vi "Autonomous Independent.vi"   [LabVIEW 2017]
doc: "This VI is called when autonomous begins, and will automatically be terminated when autonomous ends. You can carry out timed or sensor driven robot movement independently without needing to return to the caller."
uses:
  <vilib>/Rock Robotics/WPI/Utilities/WPI_GetSetVariantRefNum.vi
  <vilib>/Rock Robotics/Network Tables/NT Write Numeric Array.vi
  <vilib>/Rock Robotics/Network Tables/NT Read String.vi
  <vilib>/Rock Robotics/WPI/RobotDrive/WPI_RobotDriveMecanumDrive_Cartesian.vi
types:
  T1 = typedef "WPI_JoystickDevRef.ctl" = cluster{"Device":T2}
  T2 = typedef "WPI_JoystickDeviceEnum.ctl" = enum16{"USB 0", "USB 1", "USB 2", "USB 3", "USB 4", "USB 5"}
  T3 = typedef "WPI_RobotDriveDevRef.ctl" = cluster{"DevStatus":errorcluster, "Motors[]":T4[], "Square Inputs":bool, "Max Output":dbl}
  T4 = typedef "WPI_MotorControlDeviceRef.ctl" = cluster{"DeviceStatus":errorcluster, "Type":T5, "PWM":cluster{"PWM Channel":T6, "DeadBand":T7}, "CAN":cluster{"Device Number":u8, "SetOutput VI Ref":variant, "GetOutput VI Ref":variant, "Enable VI Ref":variant, "Disable VI Ref":variant, "Data":variant}, "Invert":bool, "DIO PWM":cluster{"PWM \"Enable\" Channel":T6, "DIOChannel":T8, "PWM Rate":dbl}}
  T5 = typedef "WPI_MotorControlType.ctl" = enum16{"PWM", "CAN", "DIO PWM"}
  T6 = typedef "FPGA_DIOPWMChannel.ctl" = enum8{"PWM 0", "PWM 1", "PWM 2", "PWM 3", "PWM 4", "PWM 5", "PWM 6", "PWM 7", "PWM 8", "PWM 9", "PWM MXP 0", "PWM MXP 1", "PWM MXP 2", "PWM MXP 3", "PWM MXP 4", "PWM MXP 5", "PWM MXP 6", "PWM MXP 7", "PWM MXP 8", "PWM MXP 9", "Invalid"}
  T7 = typedef "WPI_PWMDeadband.ctl" = cluster{"Name":string, "maxPositivePwm":i32, "minPositivePwm":i32, "centerPwm":i32, "maxNegativePwm":i32, "minNegativePwm":i32, "angularRange":u16}
  T8 = typedef "FPGA_DIOChannel.ctl" = enum8{"DIO 0", "DIO 1", "DIO 2", "DIO 3", "DIO 4", "DIO 5", "DIO 6", "DIO 7", "DIO 8", "DIO 9", "DIO MXP 0", "DIO MXP 1", "DIO MXP 2", "DIO MXP 3", "DIO MXP 4", "DIO MXP 5", "DIO MXP 6", "DIO MXP 7", "DIO MXP 8", "DIO MXP 9", "DIO MXP 10", "DIO MXP 11", "DIO MXP 12", "DIO MXP 13", "DIO MXP 14", "DIO MXP 15", "SPI Port CS1", "SPI Port CS2", "SPI Port CS3", "SPI Port MISO", "SPI Port MOSI", "Invalid"}
  T9 = typedef "WPI_GyroDevRef.ctl" = cluster{"DevStatus":errorcluster, "Analog Channel":T10, "Gain (VoltsPerDegree/Second)":dbl, "Gyro Type":enum16{"Analog", "XRS450"}, "Handle":i32, "SPI Bus":T11, "Device Found":bool, "Sample Rate":dbl, "Calibrate On Open":bool, "Offset":dbl}
  T10 = typedef "FPGA_AIChannel.ctl" = enum8{"AI 0", "AI 1", "AI 2", "AI 3", "AI MXP 0", "AI MXP 1", "AI MXP 2", "AI MXP 3", "Invalid"}
  T11 = typedef "spi_bus.ctl" = enum16{"SPI On-Board, CS0", "SPI On-Board, CS1", "SPI On-Board, CS2", "SPI On-Board, CS3", "SPI MXP", "Invalid"}
  T12 = typedef "WPI_EncoderDevRef.ctl" = cluster{"DevStatus":errorcluster, "EncoderIndex":T13, "CounterIndex":T14, "DistancePerCount":dbl, "Decoding Type":T15}
  T13 = typedef "FPGA_EncoderIdx.ctl" = enum8{"Enc 0", "Enc 1", "Enc 2", "Enc 3", "Enc 4", "Enc 5", "Enc 6", "Enc 7", "Invalid"}
  T14 = typedef "FPGA_CounterCtrSystemIndex.ctl" = enum8{"Ctr 0", "Ctr 1", "Ctr 2", "Ctr 3", "Ctr 4", "Ctr 5", "Ctr 6", "Ctr 7", "Invalid"}
  T15 = typedef "WPI_EncoderType.ctl" = enum16{"1x", "2x", "4x"}
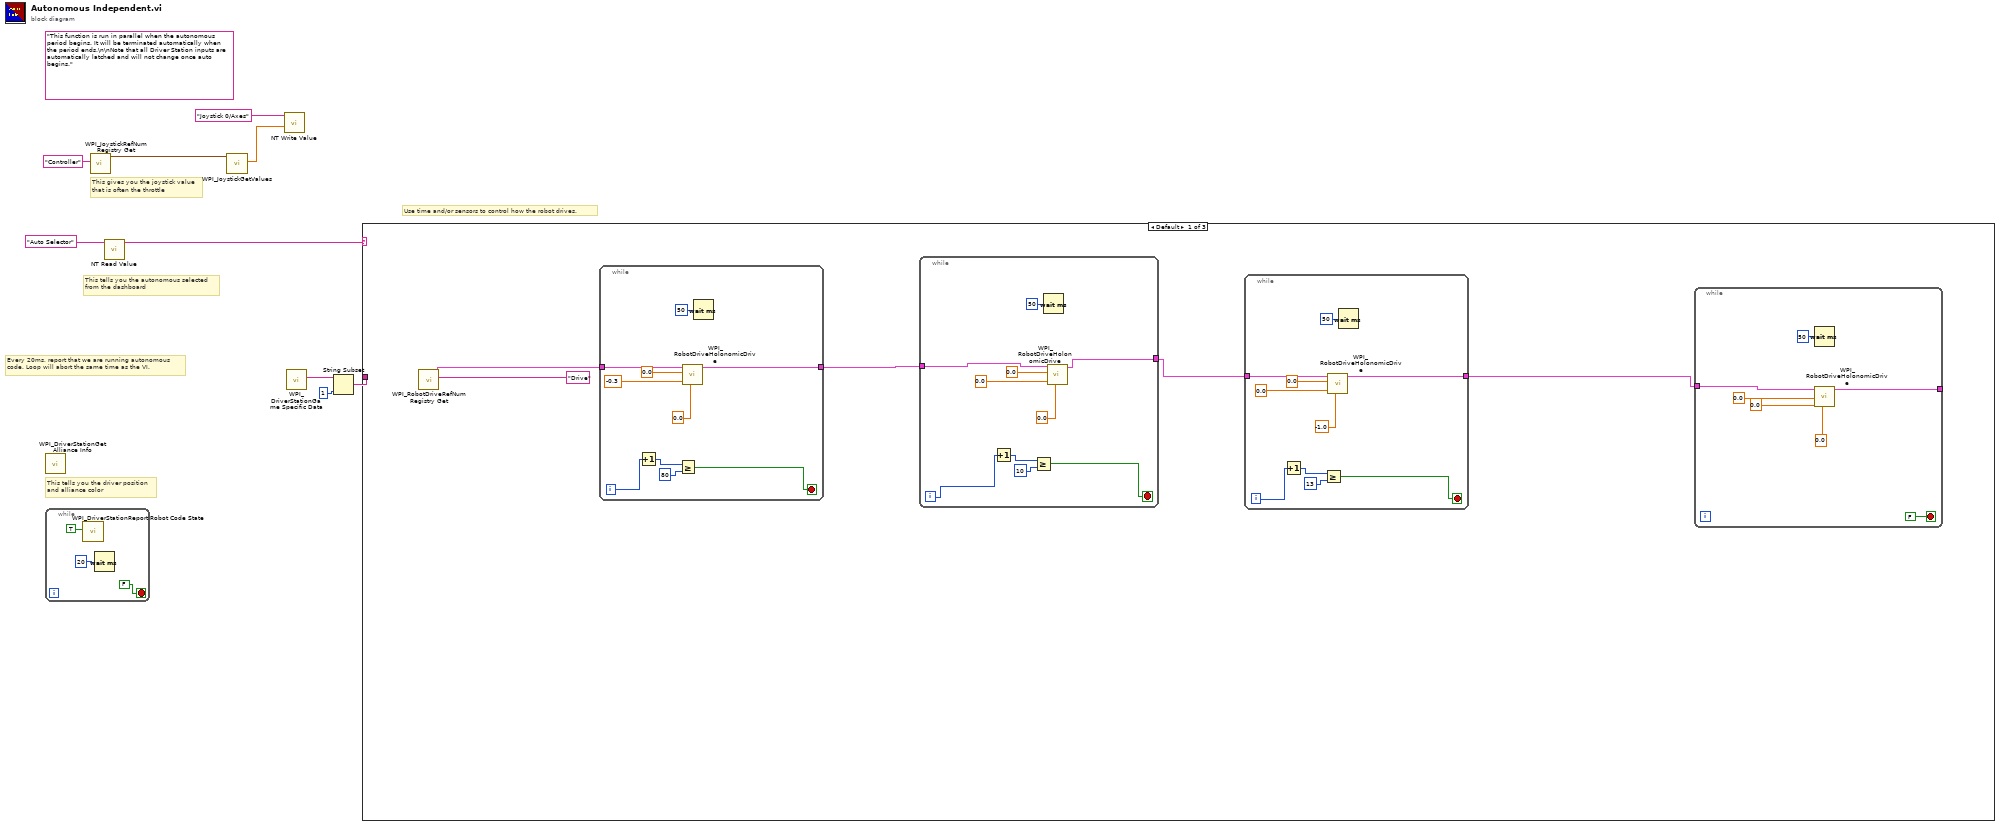
[diagram p0: block diagram]
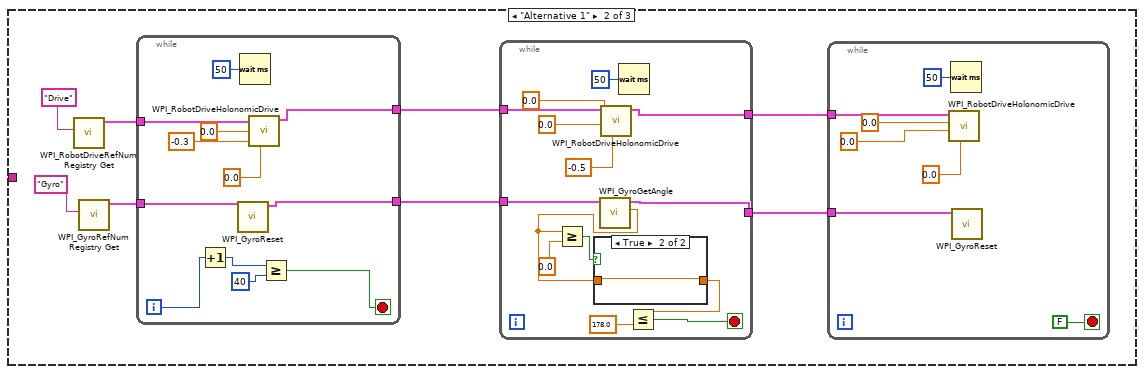
[diagram p2: hidden frame]
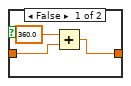
[diagram p3: hidden frame]
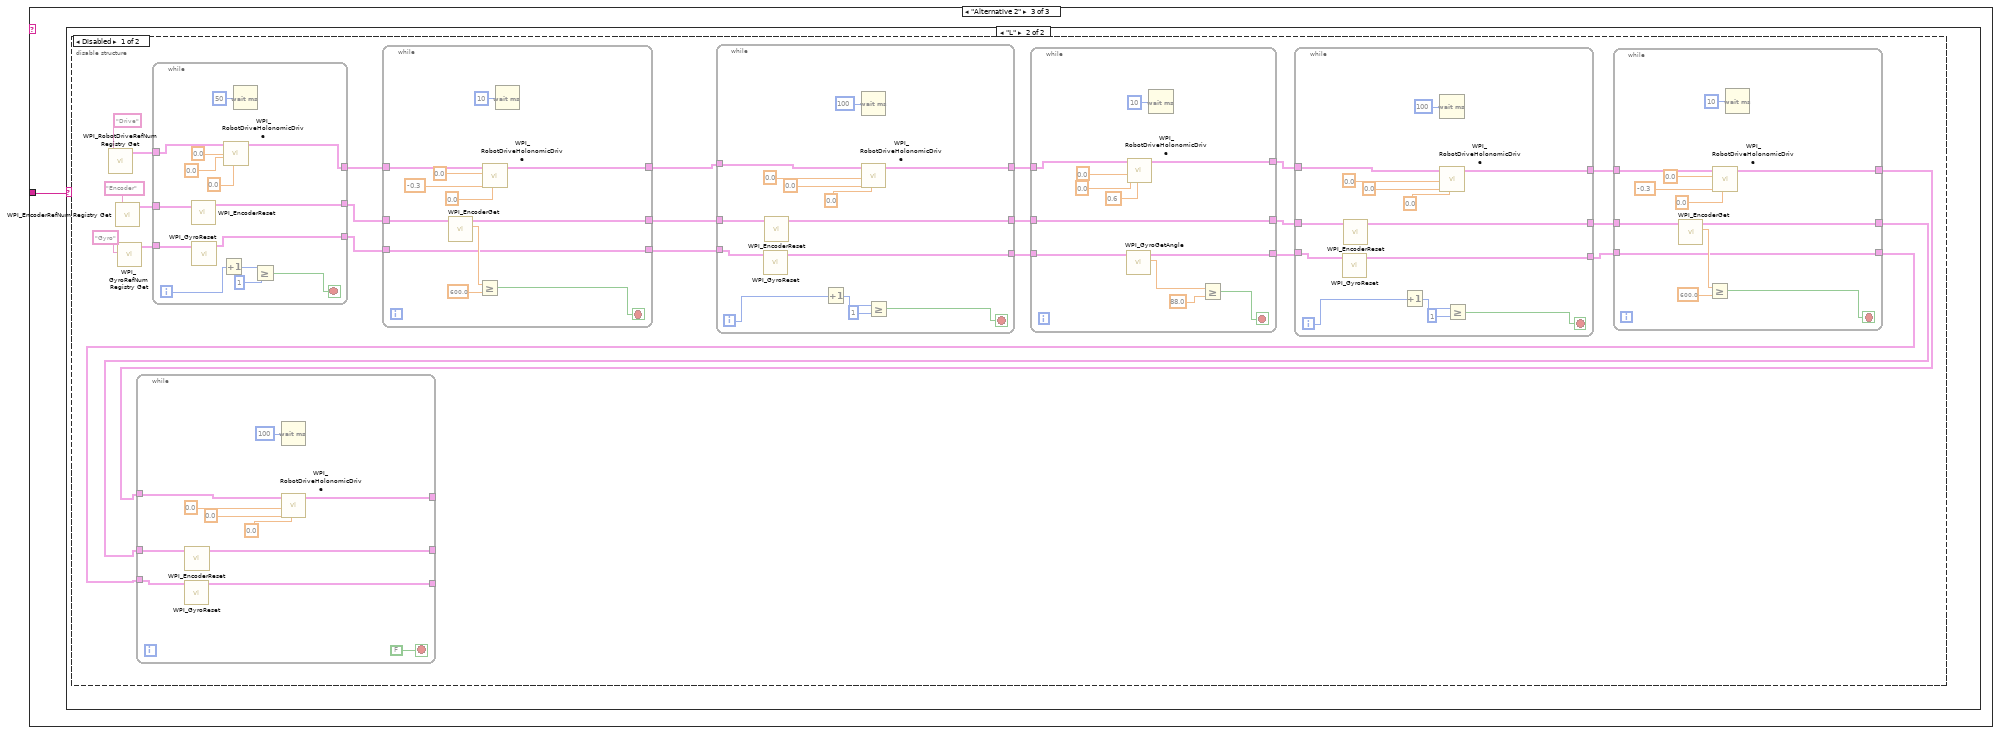
[diagram p4: hidden frame]
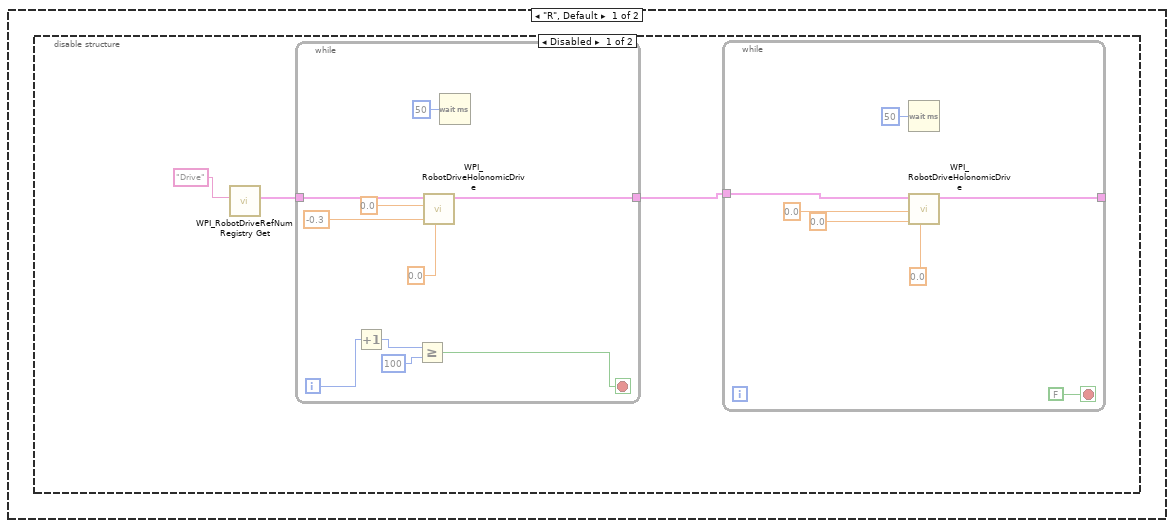
[diagram p5: hidden frame]
diagram:
  (unwired) "This function is run in parallel when the autonomous period begins. It will be terminated automatically when the period ends.\n\nNote that all Driver Station inputs are automatically latched and will not change once auto begins."
  # "This tells you the autonomous selected\nfrom the dashboard"
  # "Use time and/or sensors to control how the robot drives."
  # "Every 20ms, report that we are running autonomous\ncode. Loop will abort the same time as the VI."
  # "This gives you the joystick value\nthat is often the throttle"
  # "This tells you the driver position\nand alliance color"
  n1 = call <vilib>:"WPI_DriverStationGet Alliance Info.vi"() -> ()  [unwired: 12 out]
  n2 = while {
    stop <- FALSE stop-if-true
    n3 = call <vilib>:"WPI_DriverStationReport Robot Code State.vi"("Autonomous"=TRUE) -> ()  [unwired: 10 in, 1 out]
    n4 = Wait (ms)(milliseconds to wait=u32 20) -> ()  [unwired: 1 out]
  }
  n5 = call <vilib>:"WPI_JoystickRefNum Registry Get.vi"("refnum name"="Controller") -> ("JoystickDevRef"=w8:T1)  [unwired: 1 in, 9 out]
  n6 = call-poly <vilib>:"NT Read Value.vi"("Name"="Auto Selector") -> ("String"=w4:string)  [unwired: 9 in, 1 out]
  n7 = call <vilib>:"WPI_JoystickGetValues.vi"("JoystickDevRef"=w8) -> ("Axes"=w7:dbl[])  [unwired: 6 in, 4 out]
  n8 = call-poly <vilib>:"NT Write Value.vi"("Numeric Array"=w7, "Name"="Joystick 0/Axes") -> ()  [unwired: 9 in, 1 out]
  n9 = call <vilib>:"WPI_DriverStationGame Specific Data.vi"() -> ("Game Specific Data"=w2:string)  [unwired: 11 in]
  n10 = String Subset(string=w2, length (rest)=1 ("length (rest)")) -> (substring=w1:string)  [unwired: 1 in]
  n11 = case shown="Default" w4 {
    tunnel: w1 -> [_ _ w100]
    frame Default {
      n12 = call <vilib>:"WPI_RobotDriveRefNum Registry Get.vi"("refnum name"="Drive") -> ("RobotDriveDevRef"=w17:T3)  [unwired: 9 in, 1 out]
      n13 = while {
        tunnel: w17 -> [w54]
        tunnel: [w45] -> w15
        i -> [w49]
        stop <- w46 stop-if-true
        n14 = Increment(x=w49) -> (x+1=w48:i32)
        n15 = Greater Or Equal?(x=w48, y=80) -> (x >= y?=w46:bool)
        n16 = call-poly <vilib>:"WPI_RobotDriveHolonomicDrive.vi"("Rotation"=0.0, "Y"=-0.3, "X"=0.0, "RobotDriveDevRef"=w54) -> ("RobotDriveDevRef"=w45:T3)  [unwired: 5 in, 2 out]
        n17 = Wait (ms)(milliseconds to wait=u32 50) -> ()  [unwired: 1 out]
      }
      n18 = while {
        tunnel: w15 -> [w34]
        tunnel: [w33] -> w14
        i -> [w30]
        stop <- w29 stop-if-true
        n19 = Increment(x=w30) -> (x+1=w32:i32)
        n20 = Greater Or Equal?(x=w32, y=10) -> (x >= y?=w29:bool)
        n21 = Wait (ms)(milliseconds to wait=u32 50) -> ()  [unwired: 1 out]
        n22 = call-poly <vilib>:"WPI_RobotDriveHolonomicDrive.vi"("Rotation"=0.0, "Y"=0.0, "X"=0.0, "RobotDriveDevRef"=w34) -> ("RobotDriveDevRef"=w33:T3)  [unwired: 5 in, 2 out]
      }
      n23 = while {
        tunnel: w14 -> [w27]
        tunnel: [w18] -> w13
        i -> [w22]
        stop <- w19 stop-if-true
        n24 = Increment(x=w22) -> (x+1=w21:i32)
        n25 = Greater Or Equal?(x=w21, y=13) -> (x >= y?=w19:bool)
        n26 = call-poly <vilib>:"WPI_RobotDriveHolonomicDrive.vi"("Rotation"=-1.0, "Y"=0.0, "X"=0.0, "RobotDriveDevRef"=w27) -> ("RobotDriveDevRef"=w18:T3)  [unwired: 5 in, 2 out]
        n27 = Wait (ms)(milliseconds to wait=u32 50) -> ()  [unwired: 1 out]
      }
      n28 = while {
        tunnel: w13 -> [w44]
        tunnel: [w43] -> _
        stop <- FALSE stop-if-true
        n29 = Wait (ms)(milliseconds to wait=u32 50) -> ()  [unwired: 1 out]
        n30 = call-poly <vilib>:"WPI_RobotDriveHolonomicDrive.vi"("Rotation"=0.0, "Y"=0.0, "X"=0.0, "RobotDriveDevRef"=w44) -> ("RobotDriveDevRef"=w43:T3)  [unwired: 5 in, 2 out]
      }
    }
    frame "Alternative 1" {
      n31 = call <vilib>:"WPI_RobotDriveRefNum Registry Get.vi"("refnum name"="Drive") -> ("RobotDriveDevRef"=w62:T3)  [unwired: 9 in, 1 out]
      n32 = call <vilib>:"WPI_GyroRefNum Registry Get.vi"("refnum name"="Gyro") -> ("GyroDevRef"=w57:T9)  [unwired: 9 in, 1 out]
      n33 = while {
        tunnel: w62 -> [w99]
        tunnel: [w98] -> w61
        tunnel: w57 -> [w97]
        tunnel: [w96] -> w56
        i -> [w90]
        stop <- w89 stop-if-true
        n34 = Increment(x=w90) -> (x+1=w92:i32)
        n35 = call <vilib>:"WPI_GyroReset.vi"("GyroDevRef"=w97) -> ("GyroDevRef"=w96:T9)  [unwired: 9 in, 1 out]
        n36 = Wait (ms)(milliseconds to wait=u32 50) -> ()  [unwired: 1 out]
        n37 = call-poly <vilib>:"WPI_RobotDriveHolonomicDrive.vi"("Rotation"=0.0, "Y"=-0.3, "X"=0.0, "RobotDriveDevRef"=w99) -> ("RobotDriveDevRef"=w98:T3)  [unwired: 5 in, 2 out]
        n38 = Greater Or Equal?(x=w92, y=40) -> (x >= y?=w89:bool)
      }
      n39 = while {
        tunnel: w61 -> [w83]
        tunnel: [w82] -> w60
        tunnel: w56 -> [w81]
        tunnel: [w80] -> w55
        stop <- w78 stop-if-true
        n40 = call <vilib>:"WPI_GyroGetAngle.vi"("GyroDevRef"=w81) -> ("Angle"=w72:dbl, "GyroDevRef"=w80:T9)  [unwired: 6 in, 3 out]
        n41 = Greater Or Equal?(x=w72, y=0.0) -> (x >= y?=w73:bool)
        n42 = case shown="True" w73 {
          tunnel: [w84 w87] -> w71
          tunnel: w72 -> [w85 w87]
          frame False {
            n43 = Add(x=360.0, y=w85) -> (x+y=w84:dbl)
          }
          frame True {
          }
        }
        n44 = call-poly <vilib>:"WPI_RobotDriveHolonomicDrive.vi"("Rotation"=-0.5, "Y"=0.0, "X"=0.0, "RobotDriveDevRef"=w83) -> ("RobotDriveDevRef"=w82:T3)  [unwired: 5 in, 2 out]
        n45 = Wait (ms)(milliseconds to wait=u32 50) -> ()  [unwired: 1 out]
        n46 = Less Or Equal?(x=w71, y=178.0) -> (x <= y?=w78:bool)
      }
      n47 = while {
        tunnel: w60 -> [w69]
        tunnel: w55 -> [w68]
        stop <- FALSE stop-if-true
        n48 = call-poly <vilib>:"WPI_RobotDriveHolonomicDrive.vi"("Rotation"=0.0, "Y"=0.0, "X"=0.0, "RobotDriveDevRef"=w69) -> ()  [unwired: 5 in, 3 out]
        n49 = Wait (ms)(milliseconds to wait=u32 50) -> ()  [unwired: 1 out]
        n50 = call <vilib>:"WPI_GyroReset.vi"("GyroDevRef"=w68) -> ()  [unwired: 9 in, 2 out]
      }
    }
    frame "Alternative 2" {
      n51 = case shown="\"L\"" w100 {
        frame "R", Default {
          n52 = disable-structure shown="Disabled" {
            frame Disabled {
              n53 = call <vilib>:"WPI_RobotDriveRefNum Registry Get.vi"("refnum name"="Drive") -> ("RobotDriveDevRef"=w103:T3)  [unwired: 9 in, 1 out]
              n54 = while {
                tunnel: w103 -> [w120]
                tunnel: [w111] -> w102
                i -> [w115]
                stop <- w112 stop-if-true
                n55 = Increment(x=w115) -> (x+1=w114:i32)
                n56 = Greater Or Equal?(x=w114, y=100) -> (x >= y?=w112:bool)
                n57 = call-poly <vilib>:"WPI_RobotDriveHolonomicDrive.vi"("Rotation"=0.0, "Y"=-0.3, "X"=0.0, "RobotDriveDevRef"=w120) -> ("RobotDriveDevRef"=w111:T3)  [unwired: 5 in, 2 out]
                n58 = Wait (ms)(milliseconds to wait=u32 50) -> ()  [unwired: 1 out]
              }
              n59 = while {
                tunnel: w102 -> [w110]
                tunnel: [w109] -> _
                stop <- FALSE stop-if-true
                n60 = Wait (ms)(milliseconds to wait=u32 50) -> ()  [unwired: 1 out]
                n61 = call-poly <vilib>:"WPI_RobotDriveHolonomicDrive.vi"("Rotation"=0.0, "Y"=0.0, "X"=0.0, "RobotDriveDevRef"=w110) -> ("RobotDriveDevRef"=w109:T3)  [unwired: 5 in, 2 out]
              }
            }
            frame Enabled {
            }
          }
        }
        frame "L" {
          n62 = disable-structure shown="Disabled" {
            frame Disabled {
              n63 = call <vilib>:"WPI_RobotDriveRefNum Registry Get.vi"("refnum name"="Drive") -> ("RobotDriveDevRef"=w141:T3)  [unwired: 9 in, 1 out]
              n64 = call <vilib>:"WPI_EncoderRefNum Registry Get.vi"("refnum name"="Encoder") -> ("EncoderDevRef"=w138:T12)  [unwired: 9 in, 1 out]
              n65 = call <vilib>:"WPI_GyroRefNum Registry Get.vi"("refnum name"="Gyro") -> ("GyroDevRef"=w137:T9)  [unwired: 9 in, 1 out]
              n66 = while {
                tunnel: [w206] -> w143
                tunnel: w141 -> [w207]
                tunnel: w138 -> [w203]
                tunnel: w137 -> [w202]
                tunnel: [w201] -> w136
                tunnel: [w200] -> w135
                i -> [w197]
                stop <- w194 stop-if-true
                n67 = call <vilib>:"WPI_EncoderReset.vi"("EncoderDevRef"=w203) -> ("EncoderDevRef"=w201:T12)  [unwired: 9 in, 1 out]
                n68 = call <vilib>:"WPI_GyroReset.vi"("GyroDevRef"=w202) -> ("GyroDevRef"=w200:T9)  [unwired: 9 in, 1 out]
                n69 = Increment(x=w197) -> (x+1=w196:i32)
                n70 = call-poly <vilib>:"WPI_RobotDriveHolonomicDrive.vi"("Rotation"=0.0, "Y"=0.0, "X"=0.0, "RobotDriveDevRef"=w207) -> ("RobotDriveDevRef"=w206:T3)  [unwired: 5 in, 2 out]
                n71 = Wait (ms)(milliseconds to wait=u32 50) -> ()  [unwired: 1 out]
                n72 = Greater Or Equal?(x=w196, y=1) -> (x >= y?=w194:bool)
              }
              n73 = while {
                tunnel: w143 -> [w233]
                tunnel: [w227] -> w144
                tunnel: w136 -> [w226]
                tunnel: w135 -> [w223]
                tunnel: [w223] -> w133
                tunnel: [w222] -> w134
                stop <- w228 stop-if-true
                n74 = call <vilib>:"WPI_EncoderGet.vi"("EncoderDevRef"=w226) -> ("Distance"=w225:dbl, "EncoderDevRef"=w222:T12)  [unwired: 5 in, 4 out]
                n75 = Greater Or Equal?(x=w225, y=600.0) -> (x >= y?=w228:bool)
                n76 = call-poly <vilib>:"WPI_RobotDriveHolonomicDrive.vi"("Rotation"=0.0, "Y"=-0.3, "X"=0.0, "RobotDriveDevRef"=w233) -> ("RobotDriveDevRef"=w227:T3)  [unwired: 5 in, 2 out]
                n77 = Wait (ms)(milliseconds to wait=u32 10) -> ()  [unwired: 1 out]
              }
              n78 = while {
                tunnel: w144 -> [w221]
                tunnel: [w220] -> w132
                tunnel: w134 -> [w211]
                tunnel: w133 -> [w210]
                tunnel: [w209] -> w131
                tunnel: [w208] -> w130
                i -> [w215]
                stop <- w212 stop-if-true
                n79 = call <vilib>:"WPI_GyroReset.vi"("GyroDevRef"=w210) -> ("GyroDevRef"=w208:T9)  [unwired: 9 in, 1 out]
                n80 = call <vilib>:"WPI_EncoderReset.vi"("EncoderDevRef"=w211) -> ("EncoderDevRef"=w209:T12)  [unwired: 9 in, 1 out]
                n81 = Increment(x=w215) -> (x+1=w214:i32)
                n82 = Wait (ms)(milliseconds to wait=u32 100) -> ()  [unwired: 1 out]
                n83 = call-poly <vilib>:"WPI_RobotDriveHolonomicDrive.vi"("Rotation"=0.0, "Y"=0.0, "X"=0.0, "RobotDriveDevRef"=w221) -> ("RobotDriveDevRef"=w220:T3)  [unwired: 5 in, 2 out]
                n84 = Greater Or Equal?(x=w214, y=1) -> (x >= y?=w212:bool)
              }
              n85 = while {
                tunnel: w132 -> [w192]
                tunnel: w131 -> [w190]
                tunnel: w130 -> [w189]
                tunnel: [w191] -> w129
                tunnel: [w190] -> w128
                tunnel: [w188] -> w127
                stop <- w185 stop-if-true
                n86 = call <vilib>:"WPI_GyroGetAngle.vi"("GyroDevRef"=w189) -> ("Angle"=w187:dbl, "GyroDevRef"=w188:T9)  [unwired: 6 in, 3 out]
                n87 = call-poly <vilib>:"WPI_RobotDriveHolonomicDrive.vi"("Rotation"=0.6, "Y"=0.0, "X"=0.0, "RobotDriveDevRef"=w192) -> ("RobotDriveDevRef"=w191:T3)  [unwired: 5 in, 2 out]
                n88 = Wait (ms)(milliseconds to wait=u32 10) -> ()  [unwired: 1 out]
                n89 = Greater Or Equal?(x=w187, y=88.0) -> (x >= y?=w185:bool)
              }
              n90 = while {
                tunnel: w129 -> [w181]
                tunnel: [w180] -> w126
                tunnel: w128 -> [w171]
                tunnel: w127 -> [w170]
                tunnel: [w169] -> w125
                tunnel: [w168] -> w124
                i -> [w175]
                stop <- w172 stop-if-true
                n91 = call <vilib>:"WPI_GyroReset.vi"("GyroDevRef"=w170) -> ("GyroDevRef"=w168:T9)  [unwired: 9 in, 1 out]
                n92 = call <vilib>:"WPI_EncoderReset.vi"("EncoderDevRef"=w171) -> ("EncoderDevRef"=w169:T12)  [unwired: 9 in, 1 out]
                n93 = Increment(x=w175) -> (x+1=w174:i32)
                n94 = Wait (ms)(milliseconds to wait=u32 100) -> ()  [unwired: 1 out]
                n95 = call-poly <vilib>:"WPI_RobotDriveHolonomicDrive.vi"("Rotation"=0.0, "Y"=0.0, "X"=0.0, "RobotDriveDevRef"=w181) -> ("RobotDriveDevRef"=w180:T3)  [unwired: 5 in, 2 out]
                n96 = Greater Or Equal?(x=w174, y=1) -> (x >= y?=w172:bool)
              }
              n97 = while {
                tunnel: w126 -> [w167]
                tunnel: [w161] -> w123
                tunnel: w125 -> [w160]
                tunnel: w124 -> [w157]
                tunnel: [w157] -> w121
                tunnel: [w156] -> w122
                stop <- w162 stop-if-true
                n98 = call <vilib>:"WPI_EncoderGet.vi"("EncoderDevRef"=w160) -> ("Distance"=w159:dbl, "EncoderDevRef"=w156:T12)  [unwired: 5 in, 4 out]
                n99 = Greater Or Equal?(x=w159, y=600.0) -> (x >= y?=w162:bool)
                n100 = call-poly <vilib>:"WPI_RobotDriveHolonomicDrive.vi"("Rotation"=0.0, "Y"=-0.3, "X"=0.0, "RobotDriveDevRef"=w167) -> ("RobotDriveDevRef"=w161:T3)  [unwired: 5 in, 2 out]
                n101 = Wait (ms)(milliseconds to wait=u32 10) -> ()  [unwired: 1 out]
              }
              n102 = while {
                tunnel: w123 -> [w155]
                tunnel: [w154] -> _
                tunnel: w122 -> [w149]
                tunnel: w121 -> [w148]
                tunnel: [w147] -> _
                tunnel: [w146] -> _
                stop <- FALSE stop-if-true
                n103 = call <vilib>:"WPI_GyroReset.vi"("GyroDevRef"=w148) -> ("GyroDevRef"=w146:T9)  [unwired: 9 in, 1 out]
                n104 = call <vilib>:"WPI_EncoderReset.vi"("EncoderDevRef"=w149) -> ("EncoderDevRef"=w147:T12)  [unwired: 9 in, 1 out]
                n105 = Wait (ms)(milliseconds to wait=u32 100) -> ()  [unwired: 1 out]
                n106 = call-poly <vilib>:"WPI_RobotDriveHolonomicDrive.vi"("Rotation"=0.0, "Y"=0.0, "X"=0.0, "RobotDriveDevRef"=w155) -> ("RobotDriveDevRef"=w154:T3)  [unwired: 5 in, 2 out]
              }
            }
            frame Enabled {
            }
          }
        }
      }
    }
  }
